vi "test_Add Response ByteCount.vi"(8 "error in (no error)":errorcluster, 11 "TestCase in":refnum<class "Instrument Addon Scripting API Messages Unit Tests.lvclass">) -> (0 "error out":errorcluster, 3 "TestCase out":refnum<class "Instrument Addon Scripting API Messages Unit Tests.lvclass">)   [LabVIEW 2018, in "Instrument Addon Scripting API Messages Unit Tests.lvclass"]
uses:
  Instrument Addon Scripting API Messages Unit Tests.lvclass
  APIs/Scripting API/TypeDefs/ByteCount Response Settings.ctl
  APIs/Scripting API/TypeDefs/Linked Channel.ctl
  <vilib>/NI Veristand/Custom Device API/Custom Device Item Ref.ctl
  Addon/Addon Shared/Types/FG Control.ctl
  Addon/Addon Shared/Types/Response Parameters.ctl
  Addon/Addon Shared/Types/Linked Channel Cluster.ctl
  Addon/Addon Shared/Types/Response Wait Type.ctl
  Addon/Addon Shared/SubVIs/Constants.vi
  <vilib>/NI/NI VeriStand Advanced SysDef API/_SubVIs/SysDef.Search.GUID.vi
  <vilib>/NI Veristand/Custom Device API/NI VeriStand - Get Item Property.vi
  <vilib>/NI Veristand/Custom Device API/Get Item Property (String).vi
  <vilib>/NI Veristand/Custom Device API/Get Item Property (String Array).vi
  <vilib>/NI Veristand/Custom Device API/Get Item Property (Double).vi
  <vilib>/NI Veristand/Custom Device API/Get Item Property (U32).vi
  <vilib>/NI Veristand/Custom Device API/Get Item Property (Boolean).vi
  <vilib>/NI Veristand/Custom Device API/NI VeriStand - Set Item Property.vi
  <vilib>/NI Veristand/Custom Device API/Set Item Property (String).vi
  <vilib>/NI Veristand/Custom Device API/Set Item Property (String Array).vi
  <vilib>/NI Veristand/Custom Device API/Set Item Property (Double).vi
  <vilib>/NI Veristand/Custom Device API/Set Item Property (U32).vi
  <vilib>/NI Veristand/Custom Device API/Set Item Property (Boolean).vi
  APIs/Scripting API/Messages/Add Response - Byte Count.vi
  <vilib>/addons/_JKI Toolkits/VI Tester/TestCase.llb/TestCase.lvclass
  Instrument Addon Scripting API Test Assets/Instrument Addon Scripting API Test Assets.lvclass
  APIs/Scripting API/Instrument Addon Scripting API.lvlib
  <vilib>/NI Veristand/Custom Device API/Custom Device API.lvlib
  Addon/Addon Shared/Instrument Addon Shared.lvlib
  <vilib>/NI/NI VeriStand Advanced SysDef API/SysDef API/Advanced System Definition.lvlib
  C:/Program Files (x86)/National Instruments/LabVIEW 2018/vi.lib/addons/_JKI Toolkits/VI Tester/TestCase.llb/TestCase.lvclass
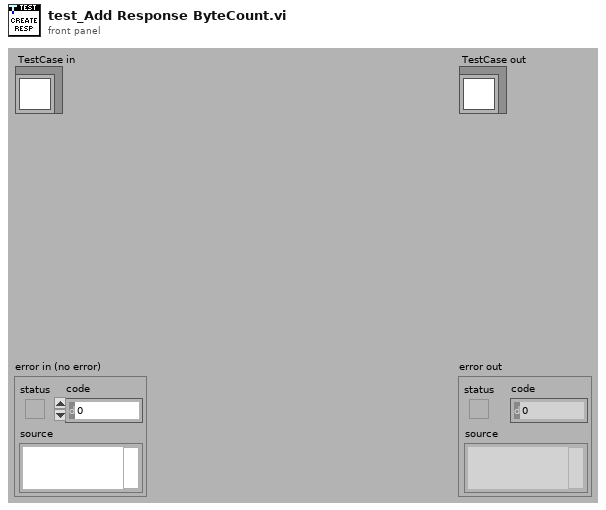
[diagram p1: front panel]
types:
  T1 = typedef "Instrument Addon Shared.lvlib/FG Control.ctl" = enum16{"Get", "Set"}
  T2 = typedef "Instrument Addon Scripting API.lvlib/ByteCount Response Settings.ctl" = cluster{"Response Format":string, "Linked Channels":T3[], "Byte Count":i32, "Use Byte Count channel":bool, "Channel Refnum":T4}
  T3 = typedef "Instrument Addon Scripting API.lvlib/Linked Channel.ctl" = cluster{"Variable Name":string, "Channel Refnum":T4}
  T4 = typedef "Custom Device API.lvlib/Custom Device Item Ref.ctl" = u64
  T5 = typedef "Instrument Addon Shared.lvlib/Response Parameters.ctl" = cluster{"Response":string, "Linked Channels":T6[], "Type Value":dbl, "Wait Type":T7, "Use Channel":bool, "Channel Path":string}
  T6 = typedef "Instrument Addon Shared.lvlib/Linked Channel Cluster.ctl" = cluster{"Variable Name":string, "GUID":string}
  T7 = typedef "Instrument Addon Shared.lvlib/Response Wait Type.ctl" = enum16{"Byte Count", "Wait sec"}
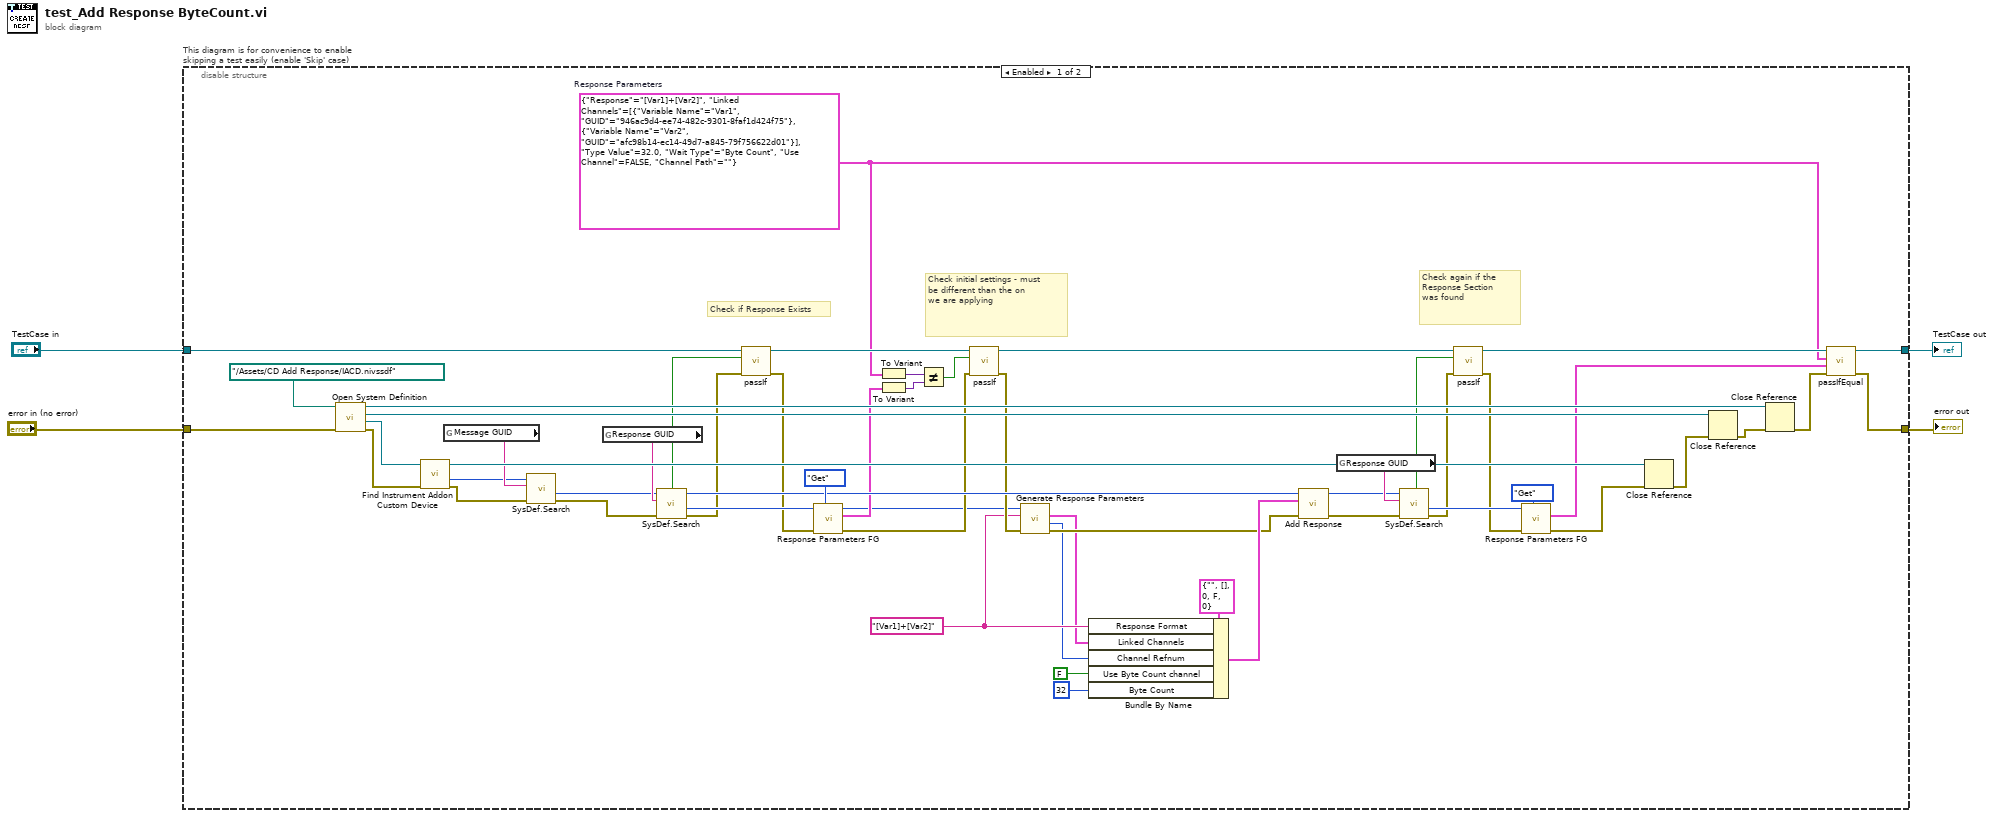
[diagram p0: block diagram]
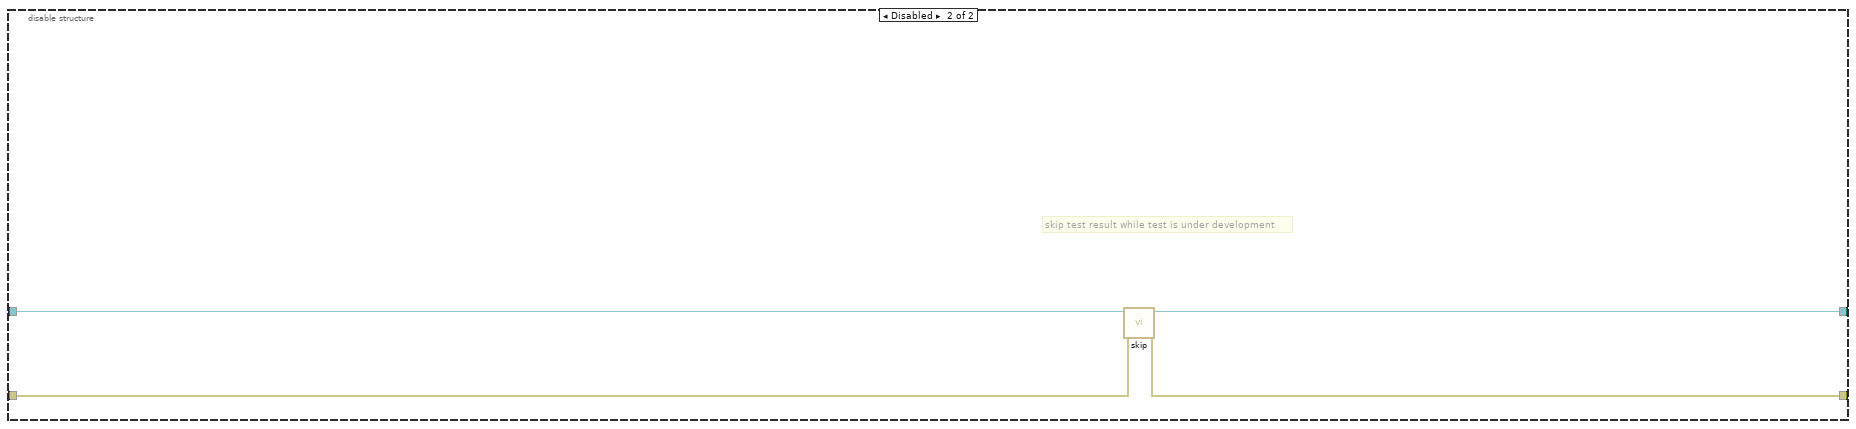
[diagram p2: hidden frame]
diagram:
  n1 = disable-structure "This diagram is for convenience to enable skipping a test easily (enable 'Skip' case)" shown="Enabled" {
    disable-tunnel: "TestCase in" -> [w29 w62]
    disable-tunnel: [w40 w60] -> w1
    disable-tunnel: [w39 w61] -> w3
    disable-tunnel: "error in (no error)" -> [w57 w59]
    frame Enabled {
      w14 = T5 {"Response"="[Var1]+[Var2]", "Linked Channels"=[{"Variable Name"="Var1", "GUID"="946ac9d4-ee74-482c-9301-8faf1d424f75"}, {"Variable Name"="Var2", "GUID"="afc98b14-ec14-49d7-a845-79f756622d01"}], "Type Value"=32.0, "Wait Type"=enum."Byte Count", "Use Channel"=FALSE, "Channel Path"=""}  # Response Parameters
      w9 = "[Var1]+[Var2]" ("Response Format")
      # "Check again if the Response Section was found"
      # "Check initial settings - must be different than the on\nwe are applying"
      # "Check if Response Exists"
      n2 = call "Open System Definition.vi"("error in (no error)"=w57, "System Definition File"=path "../Assets/CD Add Response/IACD.nivssdf" ("SDF file")) -> ("error out"=w55:errorcluster, "Target Refnum"=w54:refnum<k24>, "Root Refnum"=w53:refnum<k24>, "System Definition Refnum"=w43:refnum<k24>)  [unwired: 6 in]
      n3 = call "Find Instrument Addon Custom Device.vi"("error in"=w55, "target in"=w54) -> ("error out"=w19:errorcluster, "NodeID"=w16:u64, "target out"=w52:refnum<k24>)  [unwired: 7 in]
      n4 = global read "Constants.vi" "Message GUID"() -> (w17:string)
      n5 = call-poly <vilib>:"SysDef.Search.vi"("error in (no error)"=w19, "GUID"=w17, "nodeID"=w16) -> ("error out"=w18:errorcluster, "Value out"=w15:u64)  [unwired: 5 in, 2 out]
      n6 = global read "Constants.vi" "Response GUID"() -> (w36:string)
      n7 = call-poly <vilib>:"SysDef.Search.vi"("error in (no error)"=w18, "GUID"=w36, "nodeID"=w15) -> ("error out"=w27:errorcluster, "Value out"=w37:u64, "nodeID out"=w35:u64, "Found?"=w28:bool)  [unwired: 5 in]
      n8 = call-dynamic "passIf.vi"("error in (no error)"=w27, "pass"=w28, "TestCase in"=w29) -> ("error out"=w26:errorcluster, "TestCase out"=w25:refnum<class "Instrument Addon Scripting API Messages Unit Tests.lvclass">)  [unwired: 7 in]
      n9 = call "Response Parameters FG.vi"("Action"=FG_Control."Get", "error in (no error)"=w26, "Item Ref in"=w37) -> ("error out"=w13:errorcluster, "Response Parameters"=w34:T5, "Item Ref out"=w11:T4)  [unwired: 6 in]
      n10 = To Variant(anything=w14) -> (Variant=w33:variant)
      n11 = To Variant(anything=w34) -> (Variant=w32:variant)
      n12 = Not Equal?(x=w33, y=w32) -> (x != y?=w31:bool)
      n13 = call-dynamic "passIf.vi"("error in (no error)"=w13, "pass"=w31, "TestCase in"=w25) -> ("error out"=w12:errorcluster, "TestCase out"=w24:refnum<class "Instrument Addon Scripting API Messages Unit Tests.lvclass">)  [unwired: 7 in]
      n14 = call "Generate Response Parameters.vi"("Error In"=w12, "Response String"=w9, "Response Channel in"=w11) -> ("Error Out"=w10:errorcluster, "Wait Channel Ref out"=w7:T4, "Linked Channels"=w8:T3[])  [unwired: 5 in, 1 out]
      n15 = Bundle By Name(cluster=T2 {"Response Format"="", "Linked Channels"=[], "Byte Count"=0, "Use Byte Count channel"=FALSE, "Channel Refnum"=0} ("Settings"), "Response Format"=w9, "Linked Channels"=w8, "Channel Refnum"=w7, "Use Byte Count channel"=FALSE, "Byte Count"=32) -> (w50:T2)
      n16 = call-poly "Add Response.vi"("error in (no error)"=w10, "Settings"=w50, "Message in"=w35) -> ("error out"=w46:errorcluster, "Message out"=w45:T4)  [unwired: 7 in]
      n17 = global read "Constants.vi" "Response GUID"() -> (w47:string)
      n18 = call-poly <vilib>:"SysDef.Search.vi"("error in (no error)"=w46, "GUID"=w47, "nodeID"=w45) -> ("error out"=w23:errorcluster, "Value out"=w44:u64, "Found?"=w22:bool)  [unwired: 5 in, 1 out]
      n19 = call-dynamic "passIf.vi"("error in (no error)"=w23, "pass"=w22, "TestCase in"=w24) -> ("error out"=w21:errorcluster, "TestCase out"=w20:refnum<class "Instrument Addon Scripting API Messages Unit Tests.lvclass">)  [unwired: 7 in]
      n20 = call "Response Parameters FG.vi"("Action"=FG_Control."Get", "error in (no error)"=w21, "Item Ref in"=w44) -> ("error out"=w48:errorcluster, "Response Parameters"=w30:T5)  [unwired: 6 in, 1 out]
      n21 = Close Reference(reference=w52, error in (no error)=w48) -> (error out=w56:errorcluster)
      n22 = Close Reference(reference=w53, error in (no error)=w56) -> (error out=w42:errorcluster)
      n23 = Close Reference(reference=w43, error in (no error)=w42) -> (error out=w41:errorcluster)
      n24 = call-dynamic "passIfEqual.vi"("error in (no error)"=w41, "y"=w30, "x"=w14, "TestCase in"=w20) -> ("error out"=w39:errorcluster, "TestCase out"=w40:refnum<class "Instrument Addon Scripting API Messages Unit Tests.lvclass">)  [unwired: 6 in]
    }
    frame Disabled {
      # "skip test result while test is under development"
      n25 = call <vilib>:"skip.vi"("error in (no error)"=w59, "TestCase in"=w62) -> ("error out"=w61:errorcluster, "TestCase out"=w60:refnum<class "Instrument Addon Scripting API Messages Unit Tests.lvclass">)  [unwired: 8 in]
    }
  }
  "error out" <- w3
  "TestCase out" <- w1
